vi "SetDigitalChannelsNumber.vi"(2 "error in (no error)":errorcluster, 3 "Digital Channels":u16(ring) items=["0", "2", "4", "6", "8", "10", "12", "14", "16", "18", "20", "22", "24", "26", "28", "30", "32"], 4 "VISA resource name":refnum<visa-resource-name>) -> (0 "error out":errorcluster, 1 "VISA resource name out":refnum<visa-resource-name>)   [LabVIEW 2020, in "Active Technologies AWG3000.lvlib"]
uses:
  Active Technologies AWG3000.lvlib
panel:
  out "VISA WRITE":string
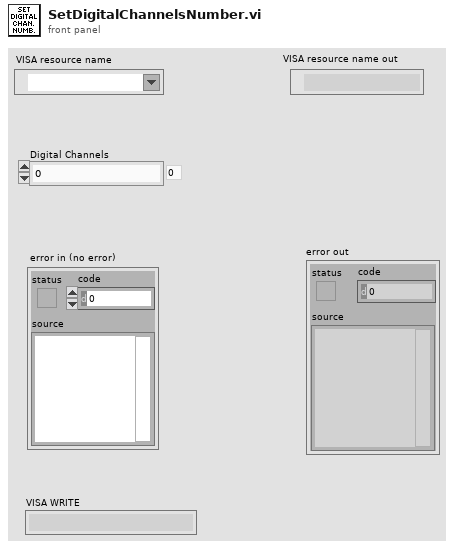
[diagram p1: front panel]
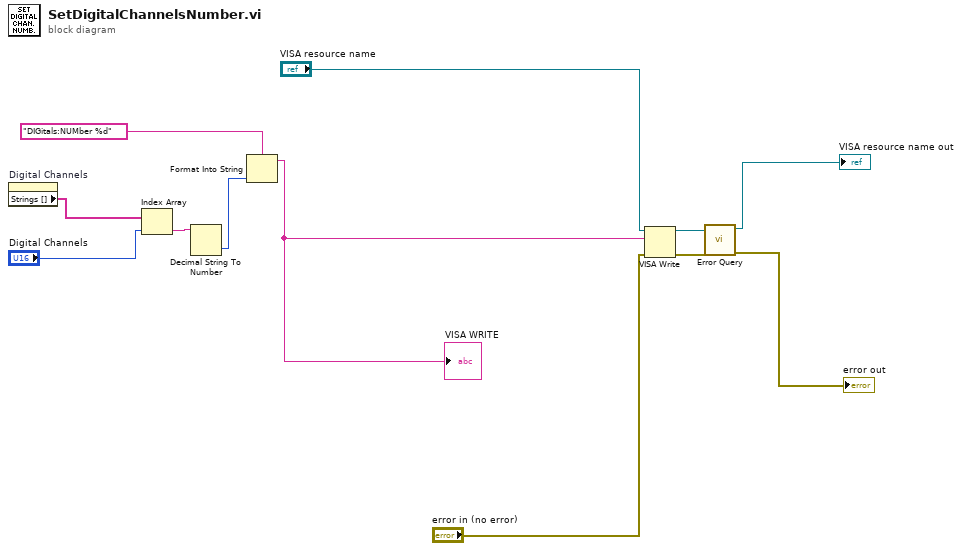
[diagram p0: block diagram]
diagram:
  n1 = property on="Digital Channels" class="Ring (strict)"() -> ("Strings []"=w5:string[])  [unwired: 2 in, 2 out]
  n2 = Index Array(array=w5, index="Digital Channels") -> (element=w3:string)
  n3 = Decimal String To Number(string=w3) -> (number=w2:i32)  [unwired: 2 in, 1 out]
  n4 = Format Into String(format string="DIGitals:NUMber %d" ("write buffer"), w2) -> (resulting string=w1:string)  [unwired: 2 in, 1 out]
  "VISA WRITE" <- w1
  n5 = VISA Write(VISA resource name="VISA resource name", write buffer=w1, error in (no error)="error in (no error)") -> (VISA resource name out=w10:refnum<visa-resource-name>, error out=w9:errorcluster)  [unwired: 1 out]
  n6 = call "Error Query.vi"("error in (no error)"=w9, "VISA resource name"=w10) -> ("error out"=→"error out":errorcluster, "VISA resource name out"=→"VISA resource name out":refnum<visa-resource-name>)  [unwired: 6 in, 2 out]
